vi "Problem 18 - Maximum path sum I.vi"(11 "Triangle of numbers":string="75\n95 64\n17 47 82\n18 35 87 10\n20 04 82 47 65\n19 01 23 75 03 34\n88 02 77 73 07 63 67\n99 65 04 28 06 16 70 92\n41 41 26 56 83 40 80 70 33\n41 48 72 33 47 32 37 16 94 29\n53 71 44 65 25 43 91 52 97 51 14\n70 11 33 28 77 73 17 78 39 68 17 57\n91 71 52 38 17 14 91 43 58 50 27 29 48\n63 66 04 68 89 53 67 30 73 16 69 87 40 31\n04 62 98 27 23 09 70 98 73 93 38 53 60 04 23") -> (1 "no. of nodes in path":i32, 2 "path":string, 3 "Answer = maximum total from top to bottom":u64, 4 "Total execution time (ms)":u32)   [LabVIEW 2021, in "Project Euler.lvlib"]
uses:
  Project Euler.lvlib
  triangle_node.ctl
  Utilities/Named Timers/Named Timers.lvlib
panel:
  out "path taken":cluster{"i":i32, "j":i32}[](array[cluster])
  out "row beneath":T1[](array[typedef])
  in  "stop early":bool
  out "row being updated":T1[](array[typedef])
  out "2D Array of nodes-being modified":T1[][](array[typedef])
  out "no. of rows":i32
  out "2D Array of nodes-initial":T1[][](array[typedef])
  out "2D Array of integers":i32[][](array[numeric])
  out "rows":string[](array[string])
  # "Input\nInputs to the VI"
  # "Development\nControls or indicators that are useful for development or testing, but which are not outputs of the VI."
  # "Output\nOutputs of the VI"
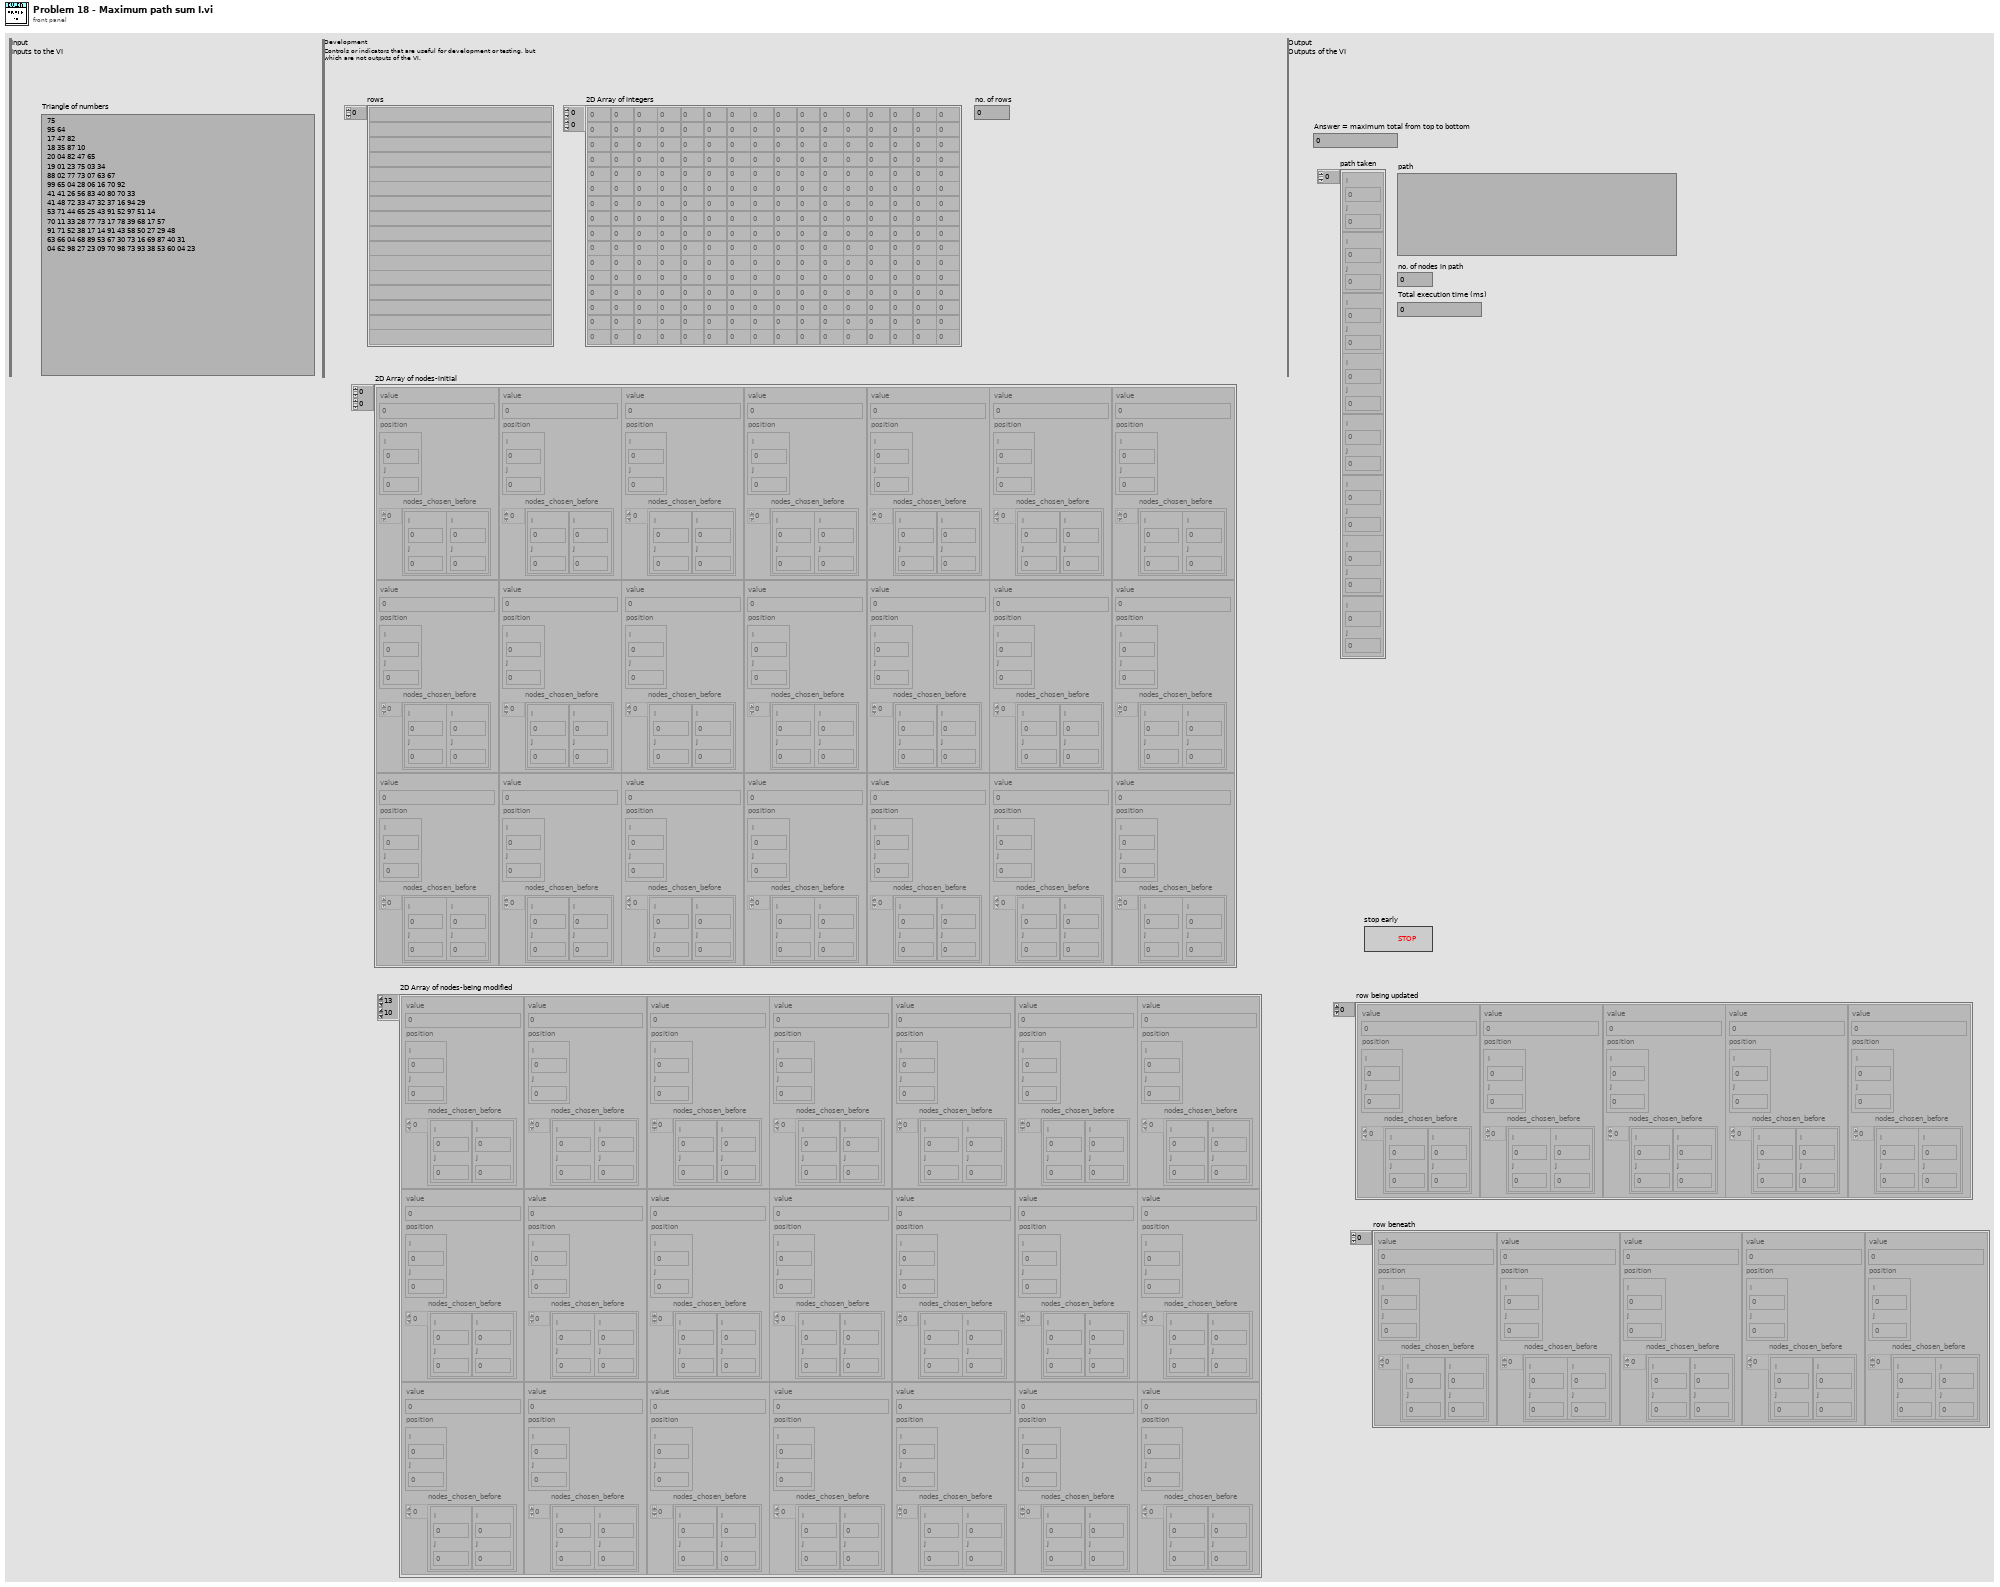
[diagram p1: front panel]
types:
  T1 = typedef "Project Euler.lvlib/triangle_node.ctl" = cluster{"value":u64, "position":cluster{"i":i32, "j":i32}, "nodes_chosen_before":cluster{"i":i32, "j":i32}[]}
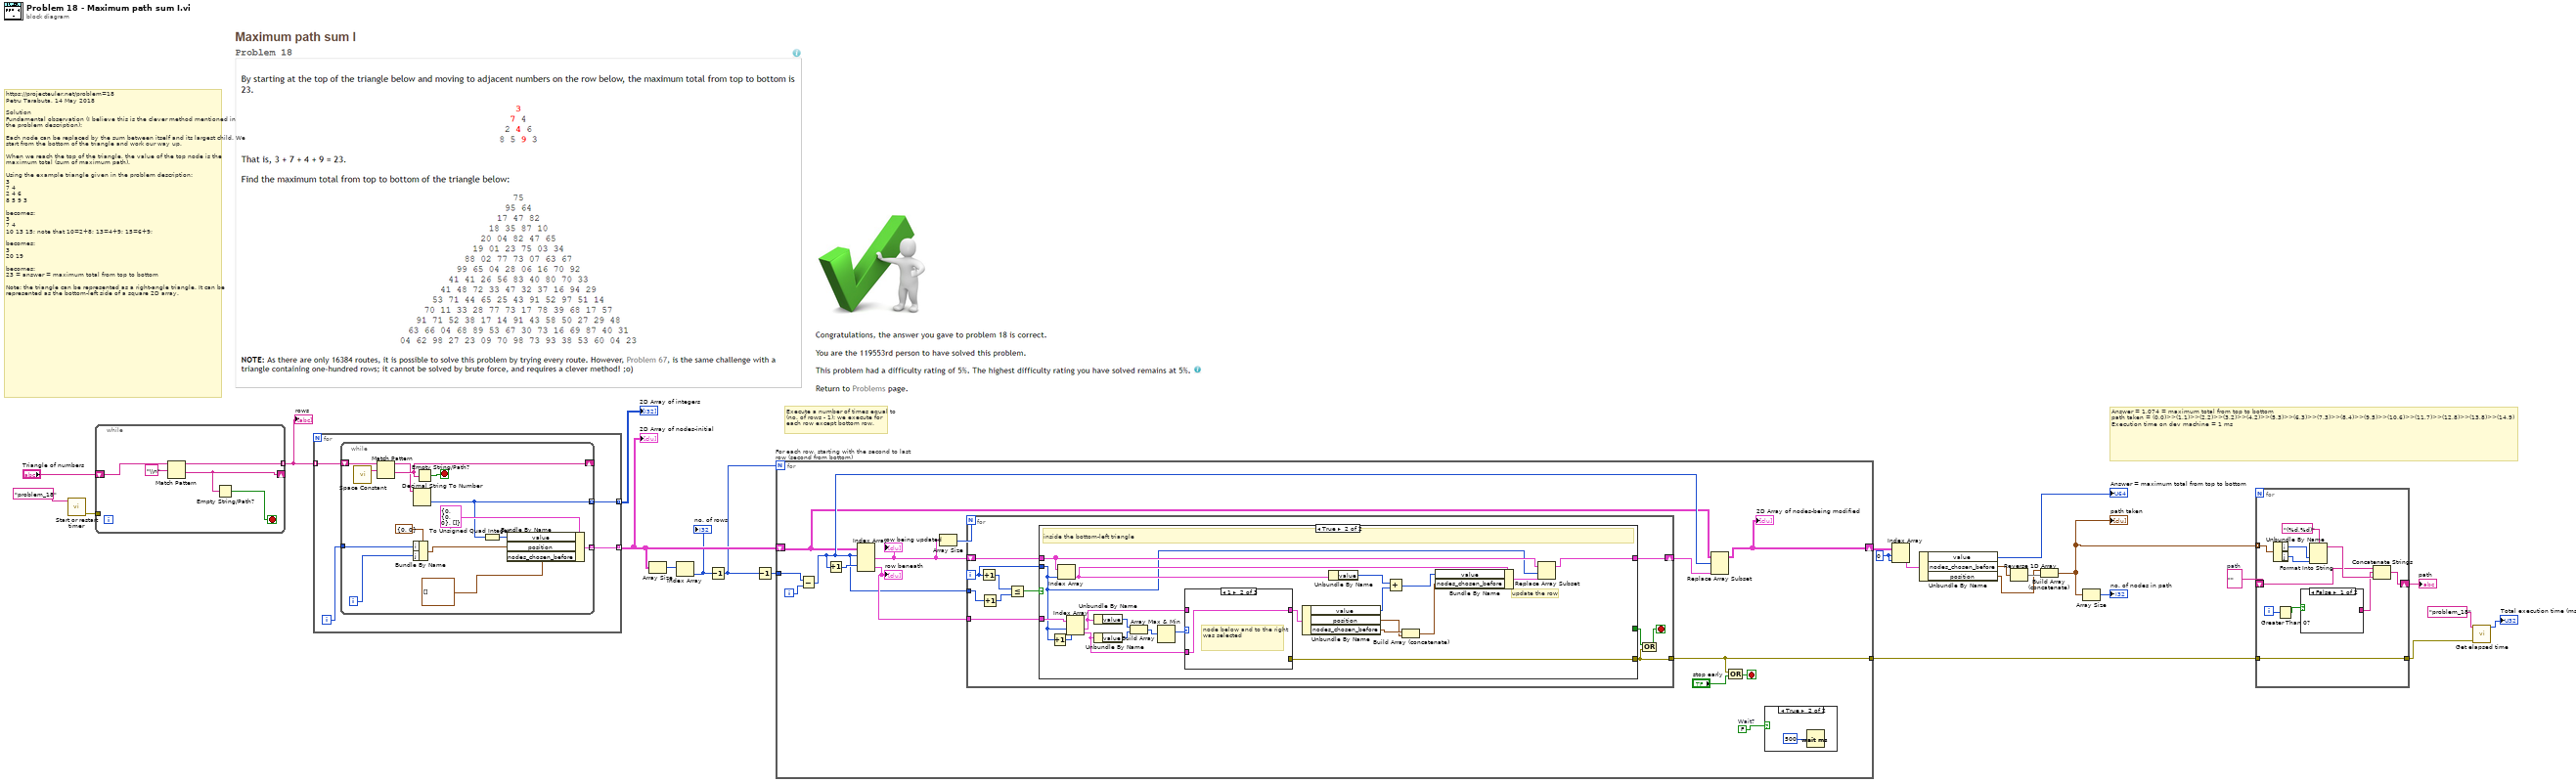
[diagram p0: block diagram]
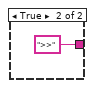
[diagram p2: hidden frame]
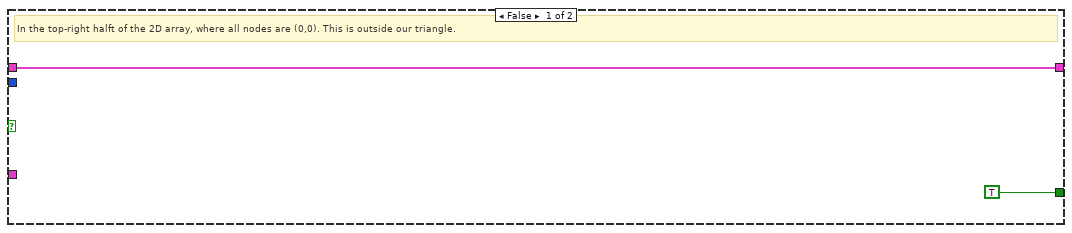
[diagram p3: hidden frame]
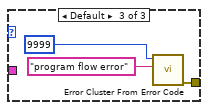
[diagram p5: hidden frame]
diagram:
  w4 = ""  # path
  w14 = 0 ("index (row)")
  # "Execute a number of times equal to (no. of rows - 1): we execute for each row except bottom row."
  # "Answer = 1,074 = maximum total from top to bottom\npath taken = (0,0)>>(1,1)>>(2,2)>>(3,2)>>(4,2)>>(5,3)>>(6,3)>>(7,3)>>(8,4)>>(9,5)>>(10,6)>>(11,7)>>(12,8)>>(13,8)>>(14,9)\nExecution time on dev machine = 1 ms"
  # "https://projecteuler.net/problem=18\nPetru Tarabuta, 14 May 2018\n\nSolution\nFundamental observation (I believe this is the clever method mentioned in the problem description):\n\nEach node can be replaced by the sum between itself and its largest child. We start from the bottom of the triangle and work our way up.\n\nWhen we reach the top of the triangle, the value of the top node is the maximum total (sum of maximum path).\n\nUsing the example triangle given in the problem description:\n3\n7 4\n2 4 6\n8 5 9 3\n\nbecomes:\n3\n7 4\n10 13 15; note that 10=2+8; 13=4+9; 15=6+9;\n\nbecomes:\n3\n20 19\n\nbecomes:\n23 = answer = maximum total from top to bottom\n\nNote: the triangle can be represented as a right-angle triangle. It can be represented as the bottom-left side of a square 2D array."
  n1 = call "Start or restart timer.vi"("Timer name"="problem_18") -> ("error out"=w7:errorcluster)  [unwired: 10 in]
  n2 = while {
    shift-right: [w27] -> _
    shift-left: "Triangle of numbers" -> [w29]
    tunnel: [w28] -> w22 mode=indexing
    tunnel: w7 -> [_]
    stop <- w26 stop-if-true
    n3 = Match Pattern(string=w29, regular expression="\\n") -> (before substring=w28:string, after substring=w27:string)  [unwired: 1 in, 2 out]
    n4 = Empty String/Path?(string/path=w27) -> (empty?=w26:bool)
  }
  "rows" <- w22
  n5 = for {
    tunnel: w22 -> [w34] mode=indexing
    tunnel: [w33] -> w21 mode=indexing
    tunnel: [w31] -> w20 mode=indexing
    i -> [w32]
    n6 = while {
      shift-right: [w46] -> _
      shift-left: w34 -> [w48]
      tunnel: [w39] -> w33 mode=indexing
      tunnel: w32 -> [w38]
      tunnel: [w35] -> w31 mode=indexing
      i -> [w37]
      stop <- w47 stop-if-true
      n7 = call <vilib>:"Space Constant.vi"() -> ("String"=w44:string)
      n8 = Match Pattern(string=w48, regular expression=w44) -> (before substring=w45:string, after substring=w46:string)  [unwired: 1 in, 2 out]
      n9 = Decimal String To Number(string=w45) -> (number=w39:i32)  [unwired: 2 in, 1 out]
      n10 = Bundle By Name(cluster=cluster{"i":i32, "j":i32} {"i"=0, "j"=0} ("position"), "i"=w38, "j"=w37) -> (w40:cluster{"i":i32, "j":i32})
      n11 = Empty String/Path?(string/path=w46) -> (empty?=w47:bool)
      n12 = To Unsigned Quad Integer(1:w39) -> (0:w36:u64)
      n13 = Bundle By Name(cluster=T1 {"value"=0, "position"={"i"=0, "j"=0}, "nodes_chosen_before"=[]} ("triangle_node"), "value"=w36, "position"=w40, "nodes_chosen_before"=cluster{"i":i32, "j":i32}[] []) -> (w35:T1)
    }
  }
  "2D Array of integers" <- w21
  "2D Array of nodes-initial" <- w20
  n14 = Array Size(array=w20) -> (size(s)=w19:i32[])
  n15 = Index Array(array=w19) -> (element=w17:i32)  [unwired: 1 in]
  "no. of rows" <- w17
  n16 = Decrement(x=w17) -> (x-1=w16:i32)
  n17 = Decrement(x=w16) -> (x-1=w18:i32)
  n18 = for "For each row, starting with the second to last row (second from bottom)" {
    N: w16 -> [_]
    shift-right: [w49] -> w15
    shift-left: w20 -> [w53]
    tunnel: w18 -> [w62]
    tunnel: [w51] -> w2
    i -> [w61]
    stop <- w50 stop-if-true
    w60 = FALSE  # Wait?
    n19 = Subtract(x=w62, y=w61) -> (x-y=w55:i32)
    n20 = Increment(x=w55) -> (x+1=w59:i32)
    n21 = Index Array(array=w53, index (row) #1=w55, index (row) #2=w59) -> (element #1=w58:T1[], element #2=w56:T1[])  [unwired: 2 in]
    "row being updated" <- w58
    "row beneath" <- w56
    n22 = Array Size(array=w58) -> (size(s)=w57:i32)
    n23 = for {
      N: w57 -> [_]
      tunnel: w55 -> [w73]
      shift-right: [w66] -> w54
      shift-left: w58 -> [w69]
      tunnel: w56 -> [w68]
      tunnel: [w63] -> w51
      i -> [w67]
      stop <- w64 stop-if-true
      n24 = Increment(x=w67) -> (x+1=w70:i32)
      n25 = Increment(x=w73) -> (x+1=w71:i32)
      n26 = Less Or Equal?(x=w70, y=w71) -> (x <= y?=w72:bool)
      n27 = case shown="True" w72 {
        tunnel: w69 -> [w74 w79]
        tunnel: w68 -> [_ w96]
        tunnel: [TRUE _] -> w65
        tunnel: w67 -> [_ w77]
        tunnel: [_ w90] -> w63
        tunnel: [w74 w76] -> w66
        frame False {
          # "In the top-right halft of the 2D array, where all nodes are (0,0). This is outside our triangle."
        }
        frame True {
          # "update the row"
          # "inside the bottom-left triangle"
          n28 = Increment(x=w77) -> (x+1=w95:i32)
          n29 = Index Array(array=w79, index=w77) -> (element=w87:T1)
          n30 = Index Array(array=w96, index #1=w77, index #2=w95) -> (element #1=w89:T1, element #2=w88:T1)
          n31 = Unbundle By Name(w89) -> ("value"=w94:u64)
          n32 = Unbundle By Name(w88) -> ("value"=w93:u64)
          n33 = Build Array(w94, w93) -> (w92:u64[])
          n34 = Array Max & Min(array=w92) -> (max index (indices)=w91:i32)  [unwired: 3 out]
          n35 = case shown="1" w91 {
            tunnel: [_ _ w101] -> w90
            tunnel: w89 -> [w97 _ _]
            tunnel: [w97 w98 _] -> w86
            tunnel: w88 -> [_ w98 _]
            frame 0 {
              # "node directly below was selected"
            }
            frame 1 {
              # "node below and to the right was selected"
            }
            frame Default {
              n36 = call <vilib>:"Error Cluster From Error Code.vi"("error message (\"\")"="program flow error" ("error message (\"\")"), "error code (0)"=9999) -> ("error out"=w101:errorcluster)  [unwired: 7 in]
            }
          }
          n37 = Unbundle By Name(w86) -> ("value"=w84:u64, "position"=w81:cluster{"i":i32, "j":i32}, "nodes_chosen_before"=w82:cluster{"i":i32, "j":i32}[])
          n38 = Unbundle By Name(w87) -> ("value"=w85:u64)
          n39 = Add(x=w85, y=w84) -> (x+y=w83:u64)
          n40 = Build Array (concatenate)(w82, w81) -> (w80:cluster{"i":i32, "j":i32}[])
          n41 = Bundle By Name(cluster=w87, "value"=w83, "nodes_chosen_before"=w80) -> (w78:T1)
          n42 = Replace Array Subset(array=w79, new element=w78, index=w77) -> (w76:T1[])
        }
      }
      n43 = Compound Arithmetic op=OR(w65, w63) -> (w64:bool)
    }
    n44 = Replace Array Subset(array=w53, new element=w54, index (row)=w55) -> (w49:T1[][])  [unwired: 1 in]
    "2D Array of nodes-being modified" <- w49
    n45 = Compound Arithmetic op=OR(w51, "stop early") -> (w50:bool)
    n46 = case shown="True" w60 {
      frame False {
      }
      frame True {
        n47 = Wait (ms)(milliseconds to wait=u32 500) -> ()  [unwired: 1 out]
      }
    }
  }
  n48 = Index Array(array=w15, index (row)=w14, index (col)=w14) -> (element=w13:T1)
  n49 = Unbundle By Name(w13) -> ("value"=→"Answer = maximum total from top to bottom":u64, "nodes_chosen_before"=w11:cluster{"i":i32, "j":i32}[], "position"=w8:cluster{"i":i32, "j":i32})
  n50 = Reverse 1D Array(array=w11) -> (reversed array=w10:cluster{"i":i32, "j":i32}[])
  n51 = Build Array (concatenate)(w8, w10) -> (w5:cluster{"i":i32, "j":i32}[])
  "path taken" <- w5
  n52 = Array Size(array=w5) -> (size(s)=→"no. of nodes in path":i32)
  n53 = for {
    tunnel: w5 -> [w113] mode=indexing
    shift-right: [w104] -> w3
    shift-left: w4 -> [w105]
    tunnel: w2 -> [w103]
    tunnel: [w103] -> w1
    i -> [w108]
    n54 = Unbundle By Name(w113) -> ("i"=w111:i32, "j"=w110:i32)
    n55 = Greater Than 0?(x=w108) -> (x > 0?=w107:bool)
    n56 = case shown="False" w107 {
      tunnel: [_ ">>"] -> w106
      frame False {
      }
      frame True {
      }
    }
    n57 = Format Into String(format string="(%d,%d)", w111, w110) -> (resulting string=w109:string)  [unwired: 2 in, 1 out]
    n58 = Concatenate Strings(w105, w106, w109) -> (w104:string)
  }
  "path" <- w3
  n59 = call "Get elapsed time.vi"("error in (no error)"=w1, "Timer name"="problem_18") -> ("Elapsed time (ms)"=→"Total execution time (ms)":u32)  [unwired: 6 in, 3 out]
